vi "Shutdown.vi"(8 "error in (no error)":errorcluster, 11 "DemoStepMotor in":refnum<class "DemoStepMotor.lvclass">) -> (0 "error out":errorcluster, 3 "DemoStepMotor out":refnum<class "DemoStepMotor.lvclass">)   [LabVIEW 2020, in "DemoStepMotor.lvlib" / "DemoStepMotor.lvclass"]
uses:
  DemoStepMotor.lvclass
  Hardware Abstraction Layer/Component/Stage/Stage/Stage.lvclass
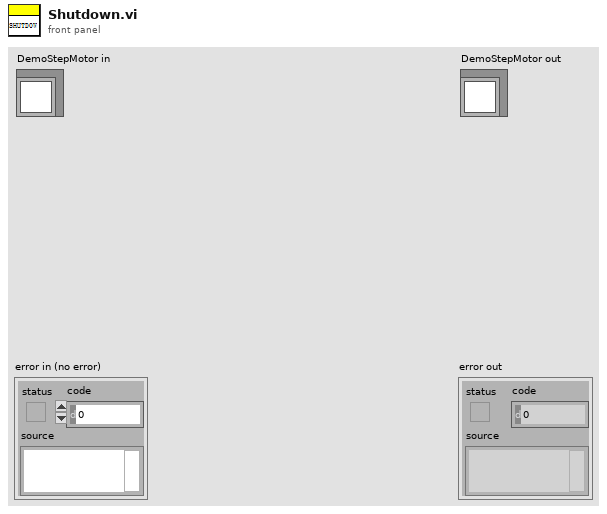
[diagram p1: front panel]
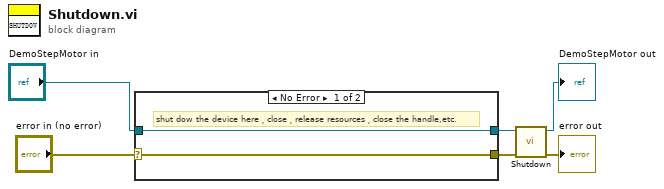
[diagram p0: block diagram]
diagram:
  n1 = case shown="No Error" "error in (no error)" {
    selector: "error in (no error)" -> [w7 w10]
    tunnel: [w7 w10] -> w2
    tunnel: [w8 w9] -> w3
    tunnel: "DemoStepMotor in" -> [w8 w9]
    frame No Error {
      # "shut dow the device here，close，release resources，close the handle,etc."
    }
    frame Error {
    }
  }
  n2 = call-parent "Shutdown.vi"("error in (no error)"=w2, "Device in"=w3) -> ("error out"=→"error out":errorcluster, "Device out"=→"DemoStepMotor out":refnum<class "DemoStepMotor.lvclass">)  [unwired: 8 in]
